vi "Catch Nested Value Update.vi"(8 "error in (no error)":errorcluster, 10 "Nested Value Update Msg":refnum<class "Nested Value Update Msg.lvclass">, 11 "ObservingViewModel In":refnum<class "ObservingViewModel.lvclass">) -> (0 "error out":errorcluster, 3 "ObservingViewModel Out":refnum<class "ObservingViewModel.lvclass">)   [LabVIEW 2017, in "TestPubSubRouting.lvlib" / "ObservingViewModel.lvclass"]
doc: "<License>\nCopyright © 2017 Composed Systems, LLC | All rights reserved\nwww.composed.io\n\nAuthor: Ethan Stern <ethan.stern@composed.io>\n\nThis software is provided \"AS IS\" WITHOUT WARRANTIES, either express or implied, AND IS FOR EDUCATIONAL PURPOSES ONLY.\n</License>"
uses:
  ObservingViewModel.lvclass
  gpm_packages/@cs/mva-viewable/Source/IViewable/IViewable Messages/Catch Nested Value Change Msg/Nested Value Update Msg.lvclass
  gpm_packages/@cs/mva-viewable/Source/IViewModel/IViewModel/IViewModel.lvclass
  C:/Git/mva-framework/Source/Framework/IViewModel/IViewModel/IViewModel.lvclass
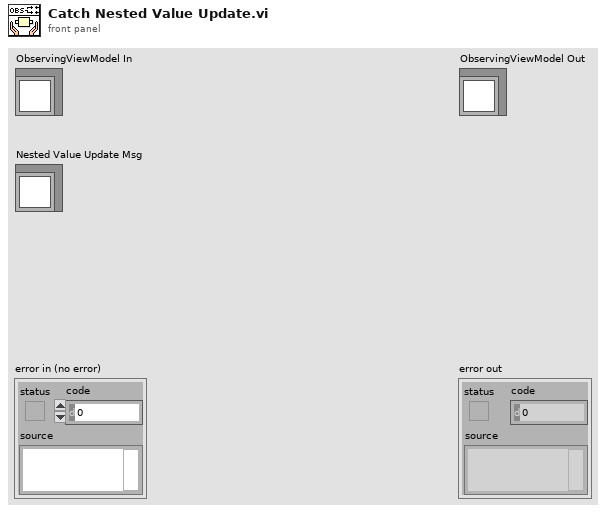
[diagram p1: front panel]
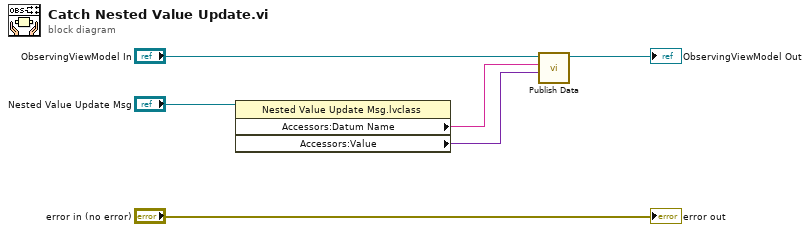
[diagram p0: block diagram]
diagram:
  n1 = property class="Nested Value Update Msg.lvclass"(reference="Nested Value Update Msg") -> ("Accessors:Datum Name"=w2:string, "Accessors:Value"=w1:variant)  [unwired: 1 in, 2 out]
  n2 = call "Publish Data.vi"("Data to Publish"=w1, "Datum Name"=w2, "IViewModel In"="ObservingViewModel In") -> ("IViewModel Out"=→"ObservingViewModel Out":refnum<class "ObservingViewModel.lvclass">)  [unwired: 7 in, 1 out]
  "error out" <- "error in (no error)"
